vi "Follow Redirect.vi"(8 "Error In":errorcluster, 11 "URL":string="https://warehouse.leapmotion.com/apps/3270/download") -> (0 "Error Out":errorcluster, 3 "URL":string)   [LabVIEW 2011, in "LMH-Toolbox.lvlib"]
uses:
  <vilib>/regexp/Match Regular Expression.xnode
  LMH-Toolbox.lvlib
  <vilib>/httpClient/LabVIEWHTTPClient.lvlib
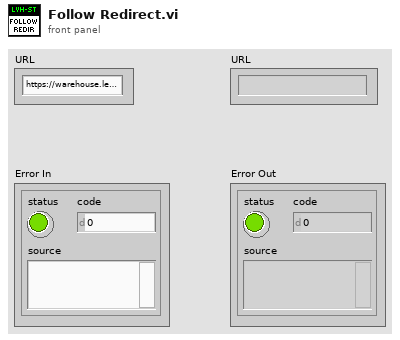
[diagram p1: front panel]
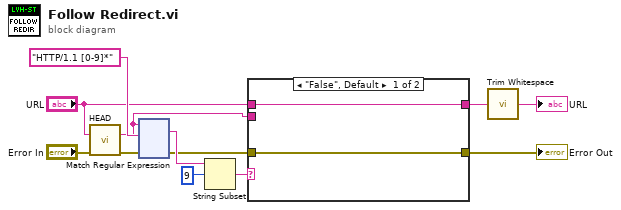
[diagram p0: block diagram]
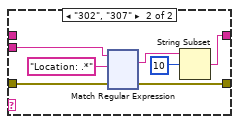
[diagram p2: hidden frame]
diagram:
  n1 = call <vilib>:"HEAD.vi"("url"="URL", "error in (no error)"="Error In") -> ("headers"=w8:string, "error out"=w4:errorcluster)  [unwired: 11 in, 1 out]
  n2 = xnode "Match Regular Expression"("input string"=w8, "regular expression"="HTTP/1.1 [0-9]*", "error in"=w4) -> ("whole match"=w11:string, "error out"=w7:errorcluster)  [unwired: 3 in, 3 out]
  n3 = String Subset(string=w11, offset (0)=9) -> (substring=w9:string)  [unwired: 1 in]
  n4 = case shown="\"False\", Default" w9 {
    tunnel: w8 -> [_ w21]
    tunnel: w7 -> [w13 w20]
    tunnel: "URL" -> [w14 _]
    tunnel: [w14 w16] -> w2
    tunnel: [w13 w15] -> w3
    frame "False", Default {
    }
    frame "302", "307" {
      n5 = xnode "Match Regular Expression"("input string"=w21, "regular expression"="Location: .*", "error in"=w20) -> ("whole match"=w17:string, "error out"=w15:errorcluster)  [unwired: 3 in, 3 out]
      n6 = String Subset(string=w17, offset (0)=10) -> (substring=w16:string)  [unwired: 1 in]
    }
  }
  "Error Out" <- w3
  n7 = call <vilib>:"Trim Whitespace.vi"("string"=w2) -> ("trimmed string"=→"URL":string)  [unwired: 1 in]
